vi "TrendStore.vi"(10 "Temperature Value":dbl, 11 "Selector":enum16{"Init", "Store", "Get"}(ring)) -> (3 "Temperature Trend":dbl[](array[numeric]))   [LabVIEW 2019, in "ControllerData.lvclass"]
uses:
  ControllerData.lvclass
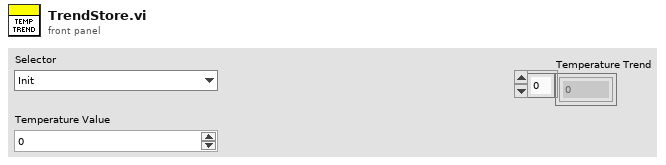
[diagram p1: front panel]
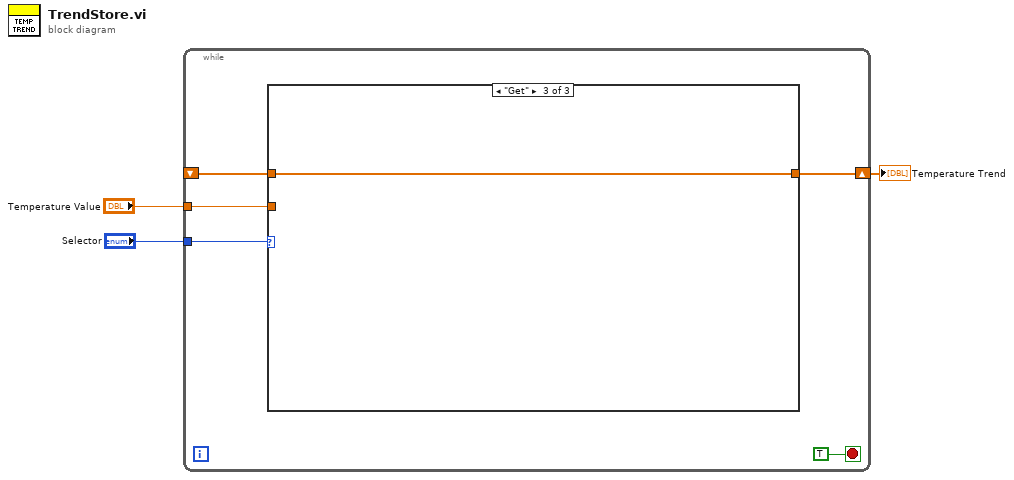
[diagram p0: block diagram]
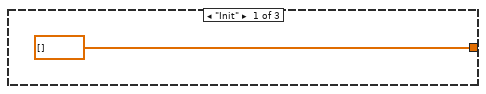
[diagram p2: hidden frame]
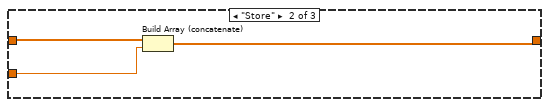
[diagram p3: hidden frame]
diagram:
  n1 = while {
    tunnel: "Selector" -> [w8]
    shift-right: [w7] -> w1
    shift-left: _ -> [w6]
    tunnel: "Temperature Value" -> [w5]
    stop <- TRUE stop-if-true
    n2 = case shown="\"Get\"" w8 {
      tunnel: [dbl[] [] w10 w13] -> w7
      tunnel: w6 -> [_ w12 w13]
      tunnel: w5 -> [_ w11 _]
      frame "Init" {
      }
      frame "Store" {
        n3 = Build Array (concatenate)(w12, w11) -> (w10:dbl[])
      }
      frame "Get" {
      }
    }
  }
  "Temperature Trend" <- w1
